vi "20170328-lecture3-bubble sort.vi"() -> ()   [LabVIEW 2014]
panel:
  out "after bubble sort":dbl[](array[numeric])
  out "before bubble sort":dbl[](array[numeric])
  out "Waveform Chart":dbl[](graph)
  # "Bubble sort is a comparison in each pair of adjacent items.\nSwap them if they are in the wrong order and pass through the list is\nrepeated until no swaps are needed\ne.g. (51428)\n(51428) > (15428)\n(15428) > (14528)\n(14529) > (14258)\n(14258) -> (14258)\n(14258) > (12458)\n\ntotal : 1024 integer numbers from  0 ~ 10,000, use Random \ngenerator, waveform graph"
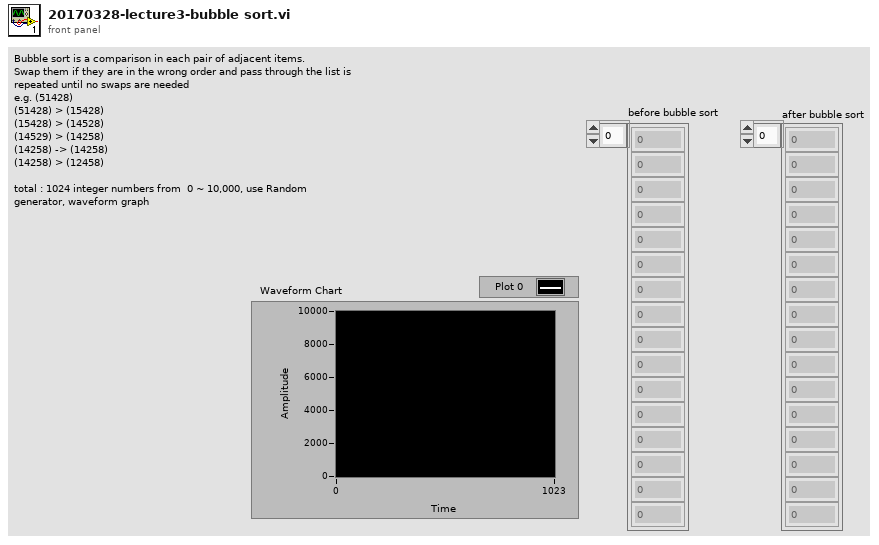
[diagram p1: front panel]
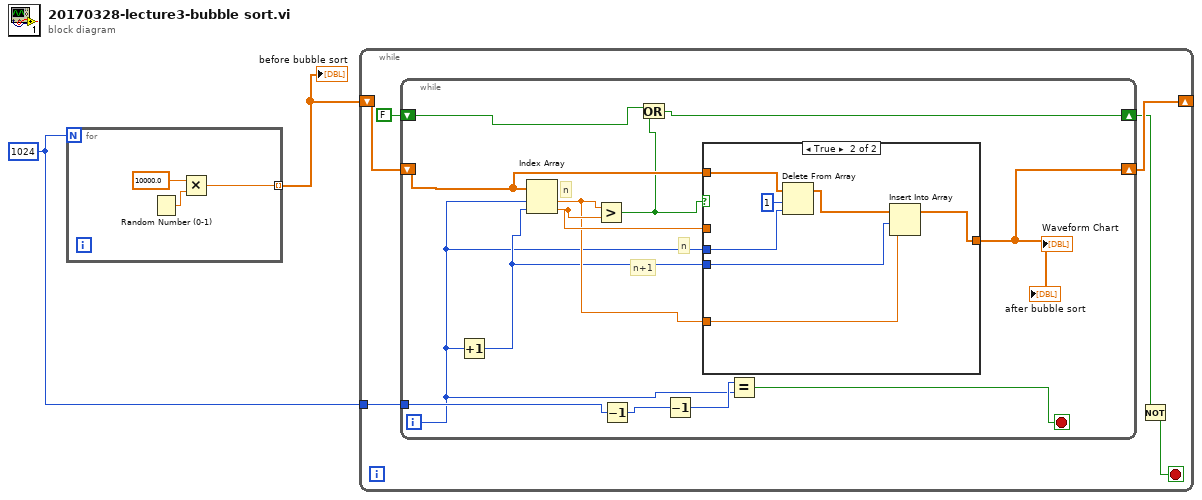
[diagram p0: block diagram]
diagram:
  w1 = 1024
  n1 = for {
    N: w1 -> [_]
    tunnel: [w3] -> w2 mode=indexing
    n2 = Random Number (0-1)() -> (number: 0 to 1=w5:dbl)
    n3 = Multiply(x=10000.0, y=w5) -> (x*y=w3:dbl)
  }
  "before bubble sort" <- w2
  n4 = while {
    tunnel: w1 -> [w10]
    shift-right: [w9] -> _
    shift-left: w2 -> [w11]
    stop <- w8 stop-if-true
    n5 = while {
      tunnel: w10 -> [w17]
      shift-right: [w15] -> w9
      shift-left: w11 -> [w24]
      shift-right: [w12] -> w7
      shift-left: FALSE -> [w13]
      i -> [w16]
      stop <- w20 stop-if-true
      # "n+1"
      # "n"
      # "n"
      n6 = Increment(x=w16) -> (x+1=w21:i32)
      n7 = Index Array(array=w24, index #1=w16, index #2=w21) -> (element #1=w22:dbl, element #2=w23:dbl)
      n8 = Greater?(x=w22, y=w23) -> (0:w14:bool)
      n9 = Decrement(x=w17) -> (x-1=w19:i32)
      n10 = Or(x=w13, y=w14) -> (x .or. y?=w12:bool)
      n11 = Decrement(x=w19) -> (x-1=w18:i32)
      n12 = case shown="True" w14 {
        tunnel: w24 -> [w25 w32]
        tunnel: w16 -> [_ w30]
        tunnel: w21 -> [_ w28]
        tunnel: w23 -> [_ _]
        tunnel: w22 -> [_ w27]
        tunnel: [w25 w26] -> w15
        frame False {
        }
        frame True {
          n13 = Delete From Array(array=w32, length=1, index=w30) -> (array with subset deleted=w29:dbl[])  [unwired: 1 out]
          n14 = Insert Into Array(array=w29, index=w28, new element=w27) -> (w26:dbl[])
        }
      }
      "Waveform Chart" <- w15
      "after bubble sort" <- w15
      n15 = Equal?(x=w18, y=w16) -> (x = y?=w20:bool)
    }
    n16 = Not(x=w7) -> (.not. x?=w8:bool)
  }
